vi "Untitled 4.vi"() -> ()   [LabVIEW 2019, in "Git.lvclass"]
uses:
  Git/Git.lvclass
  <vilib>/JKI/VIPM API/VIPM API_vipm_api.lvlib
  VIPM/VIPM.lvclass
panel:
  in  "error in (no error)":errorcluster
  in  "Git.lvclass":refnum<class "Git.lvclass">
  out "input cluster":refnum<class "Git.lvclass">
  in  "Build Path":path
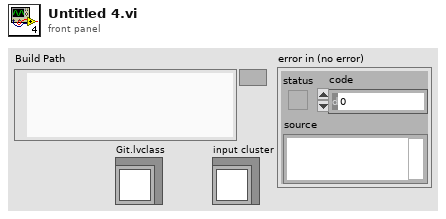
[diagram p1: front panel]
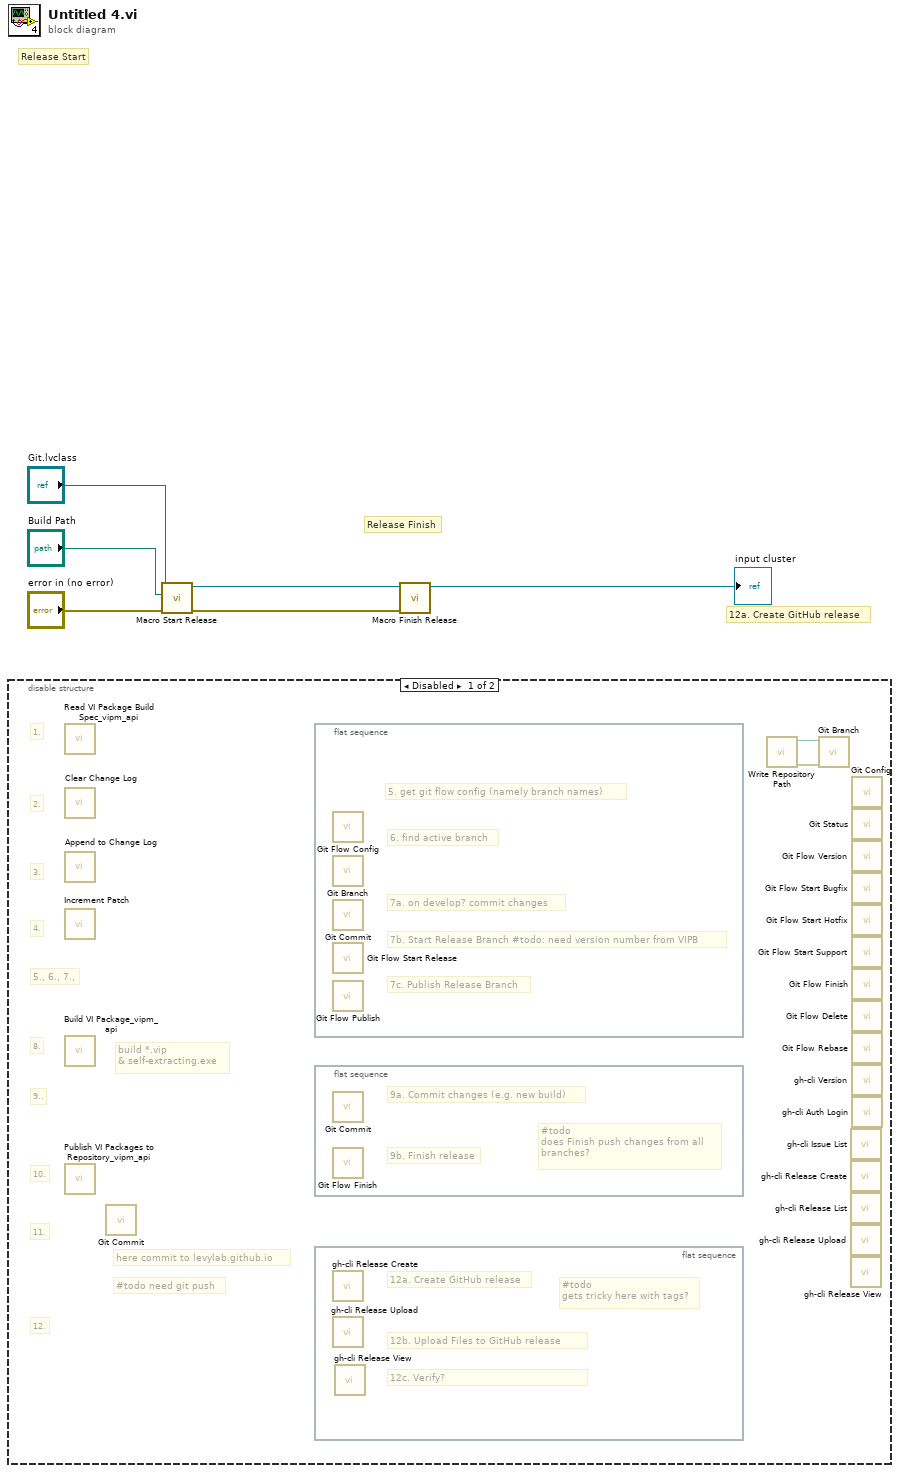
[diagram p0: block diagram]
diagram:
  # "12a. Create GitHub release"
  # "Release Finish"
  # "Release Start"
  n1 = disable-structure shown="Disabled" {
    frame Disabled {
      # "build *.vip\n& self-extracting.exe"
      # "11."
      # "10."
      # "8."
      # "3."
      # "2."
      # "4."
      # "1."
      # "#todo need git push"
      # "here commit to levylab.github.io"
      # "12."
      # "9.."
      # "5., 6., 7.,"
      n2 = call <vilib>:"Read VI Package Build Spec_vipm_api.vi"() -> ()  [unwired: 10 in, 2 out]
      n3 = call "Clear Change Log.vi"() -> ()  [unwired: 10 in, 2 out]
      n4 = call "Append to Change Log.vi"() -> ()  [unwired: 10 in, 2 out]
      n5 = call "Increment Patch.vi"() -> ()  [unwired: 10 in, 2 out]
      n6 = call <vilib>:"Build VI Package_vipm_api.vi"() -> ()  [unwired: 10 in, 2 out]
      n7 = call <vilib>:"Publish VI Packages to Repository_vipm_api.vi"() -> ()  [unwired: 10 in, 2 out]
      n8 = call "Git Commit.vi"() -> ()  [unwired: 9 in, 3 out]
      n9 = flat-sequence {
        frame #0 {
          # "7c. Publish Release Branch"
          # "7b. Start Release Branch #todo: need version number from VIPB"
          # "7a. on develop? commit changes"
          # "6. find active branch"
          # "5. get git flow config (namely branch names)"
          n10 = call "Git Flow Config.vi"() -> ()  [unwired: 9 in, 3 out]
          n11 = call "Git Branch.vi"() -> ()  [unwired: 8 in, 4 out]
          n12 = call "Git Commit.vi"() -> ()  [unwired: 9 in, 3 out]
          n13 = call "Git Flow Start Release.vi"() -> ()  [unwired: 9 in, 3 out]
          n14 = call "Git Flow Publish.vi"() -> ()  [unwired: 9 in, 3 out]
        }
      }
      n15 = flat-sequence {
        frame #0 {
          # "#todo\ndoes Finish push changes from all\nbranches?"
          # "9a. Commit changes (e.g. new build)"
          # "9b. Finish release"
          n16 = call "Git Commit.vi"() -> ()  [unwired: 9 in, 3 out]
          n17 = call "Git Flow Finish.vi"() -> ()  [unwired: 9 in, 3 out]
        }
      }
      n18 = flat-sequence {
        frame #0 {
          # "12c. Verify?"
          # "#todo\ngets tricky here with tags?"
          # "12a. Create GitHub release"
          # "12b. Upload Files to GitHub release"
          n19 = call "gh-cli Release Create.vi"() -> ()  [unwired: 10 in, 2 out]
          n20 = call "gh-cli Release Upload.vi"() -> ()  [unwired: 9 in, 3 out]
          n21 = call "gh-cli Release View.vi"() -> ()  [unwired: 9 in, 3 out]
        }
      }
      n22 = call "Write Repository Path.vi"() -> ("error out"=w8:errorcluster, "Git out"=w7:refnum<class "Git.lvclass">)  [unwired: 10 in]
      n23 = call "Git Branch.vi"("error in (no error)"=w8, "Git in"=w7) -> ()  [unwired: 6 in, 4 out]
      n24 = call "gh-cli Issue List.vi"() -> ()  [unwired: 9 in, 3 out]
      n25 = call "gh-cli Release Create.vi"() -> ()  [unwired: 10 in, 2 out]
      n26 = call "gh-cli Release List.vi"() -> ()  [unwired: 9 in, 3 out]
      n27 = call "gh-cli Release Upload.vi"() -> ()  [unwired: 9 in, 3 out]
      n28 = call "gh-cli Release View.vi"() -> ()  [unwired: 9 in, 3 out]
      n29 = call "Git Config.vi"() -> ()  [unwired: 9 in, 3 out]
      n30 = call "Git Status.vi"() -> ()  [unwired: 9 in, 3 out]
      n31 = call "Git Flow Version.vi"() -> ()  [unwired: 9 in, 3 out]
      n32 = call "Git Flow Start Bugfix.vi"() -> ()  [unwired: 9 in, 3 out]
      n33 = call "Git Flow Start Hotfix.vi"() -> ()  [unwired: 9 in, 3 out]
      n34 = call "Git Flow Start Support.vi"() -> ()  [unwired: 9 in, 3 out]
      n35 = call "Git Flow Finish.vi"() -> ()  [unwired: 9 in, 3 out]
      n36 = call "Git Flow Delete.vi"() -> ()  [unwired: 9 in, 3 out]
      n37 = call "Git Flow Rebase.vi"() -> ()  [unwired: 9 in, 3 out]
      n38 = call "gh-cli Version.vi"() -> ()  [unwired: 9 in, 3 out]
      n39 = call "gh-cli Auth Login.vi"() -> ()  [unwired: 10 in, 2 out]
    }
    frame Enabled {
    }
  }
  n40 = call "Macro Start Release.vi"("error in (no error)"="error in (no error)", "VIPB Path"="Build Path", "Git in"="Git.lvclass") -> ("error out"=w5:errorcluster, "Git out"=w3:refnum<class "Git.lvclass">)  [unwired: 7 in]
  n41 = call "Macro Finish Release.vi"("error in (no error)"=w5, "Git in"=w3) -> ("Git out"=→"input cluster":refnum<class "Git.lvclass">)  [unwired: 8 in, 1 out]
